vi "Save Logs.vi"(8 "Error In":errorcluster, 11 "EventLog in":refnum<class "ErrorLog.lvclass">) -> (0 "Error Out":errorcluster, 3 "EventLog out":refnum<class "ErrorLog.lvclass">)   [LabVIEW 2019, in "ErrorLog.lvlib" / "ErrorLog.lvclass"]
uses:
  ErrorLog.lvclass
  C:/Projekty/_Wewnetrzne/PC_ActorFramework/07_Program/LABVIEW/02_Source/SubModules/LogsAbstract/LogsAbstract.lvclass
  ErrorLog.lvclass/ErrorLog.ctl
  LogsAbstract/LogsAbstract.lvclass/LogsAbstract.ctl
  ca23ac51-5c7a-4fe6-92d9-5bdbf4829226.vi
  443144cd-2b79-43cd-aa80-fa5ab32d1dd7.vi
  1f3a0861-d62e-4685-b41d-5f2c24ac586b.vi
  1f3a0861-d62e-4685-b41d-5f2c24ac586b.vi/d883c4ce-205c-40cc-8a95-d774a9241dcb.vi
  LogsAbstract/Accessors/Write LogPath.vi
  LogsAbstract/Accessors/Read LogPath.vi
  Classes/Error/Error.lvclass
  C:/Projekty/_Wewnetrzne/PC_ActorFramework/07_Program/LABVIEW/02_Source/Classes/EventsAbstract/EventsAbstract.lvclass
  <vilib>/Utility/Data Type/Get Numeric Information.vi
  <vilib>/Utility/file.llb/Write Delimited Spreadsheet.vi
  <vilib>/Utility/file.llb/Write Delimited Spreadsheet (string).vi
  Classes/EventsAbstract/EventsAbstract.lvclass
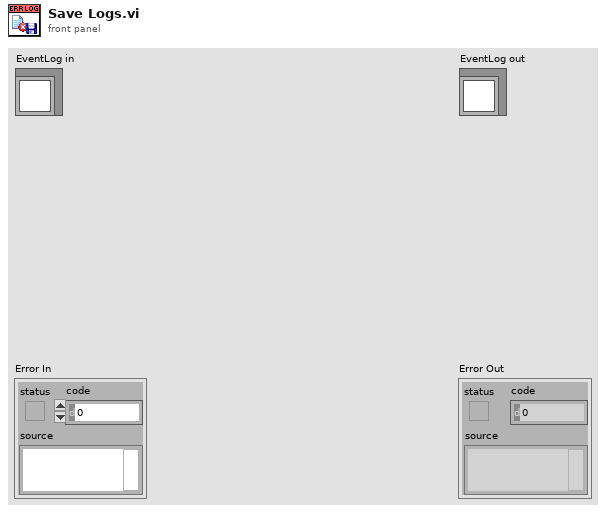
[diagram p1: front panel]
types:
  T1 = cluster{"Date":string, "Time":string, "Description":string, "Comments":string, "Source":string}
  T2 = typedef "Error.lvclass/Error Classification.ctl" = enum16{"System Error", "Process Error", "Warning", "LabView built-in"}
  T3 = cluster{"Error?":bool, "Error Code":i32, "Classification":T2, "Call Chain":string}
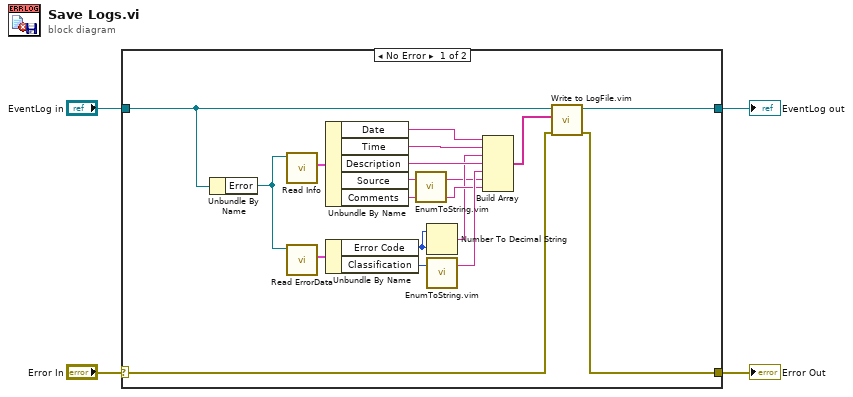
[diagram p0: block diagram]
diagram:
  n1 = case shown="No Error" "Error In" {
    selector: "Error In" -> [w20 w24]
    tunnel: [w19 w24] -> w4
    tunnel: [w21 w23] -> w3
    tunnel: "EventLog in" -> [w22 w23]
    frame No Error {
      n2 = Unbundle By Name(w22) -> ("Error"=w17:refnum<class "Error.lvclass">)
      n3 = call "Read Info.vi"("EventsAbstract in"=w17) -> ("Info"=w16:T1)  [unwired: 8 in, 2 out]
      n4 = call "Read ErrorData.vi"("Error in"=w17) -> ("ErrorData"=w15:T3)  [unwired: 8 in, 2 out]
      n5 = Unbundle By Name(w16) -> ("Date"=w13:string, "Time"=w12:string, "Description"=w11:string, "Source"=w9:string, "Comments"=w8:string)
      n6 = Unbundle By Name(w15) -> ("Error Code"=w6:i32, "Classification"=w14:T2)
      n7 = call "EnumToString.vim"("Enum"=w9) -> ("Enum Value"=w5:string)  [unwired: 16 in, 2 out]
      n8 = Number To Decimal String(number=w6, width (-)=w6) -> (decimal integer string=w7:string)
      n9 = call "EnumToString.vim"("Enum"=w14) -> ("Enum Value"=w10:string)  [unwired: 16 in, 2 out]
      n10 = Build Array(w13, w12, w7, w11, w10, w5, w8) -> (w18:string[])
      n11 = call "Write to LogFile.vim"("Error In"=w20, "Data"=w18, "LogClass In"=w22) -> ("Error out"=w19:errorcluster, "LogClass Out"=w21:refnum<class "ErrorLog.lvclass">)  [unwired: 7 in]
    }
    frame Error {
    }
  }
  "Error Out" <- w4
  "EventLog out" <- w3
